vi "Measure.vi"(8 "error in (no error)":errorcluster, 11 "IV_meas in":refnum<class "IV_meas.lvclass">) -> (0 "error out":errorcluster, 1 "Current Value":dbl, 2 "Result":dbl, 3 "IV_meas out":refnum<class "IV_meas.lvclass">)   [LabVIEW 2018, in "IV_meas.lvclass"]
uses:
  IV_meas.lvclass
  Abstract/Measurement/Measurement2D/Measurement2D.lvclass
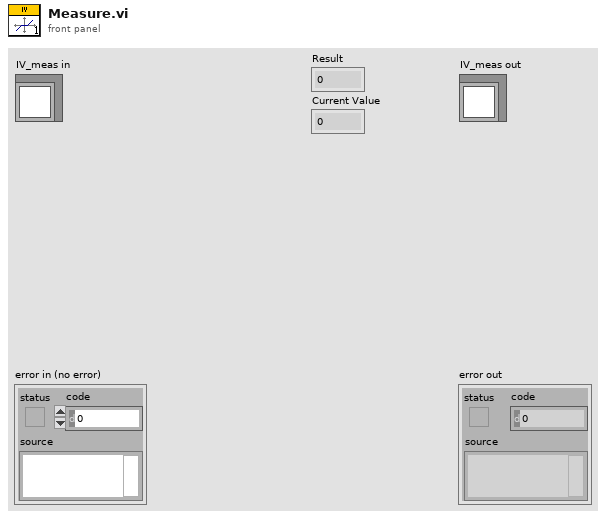
[diagram p1: front panel]
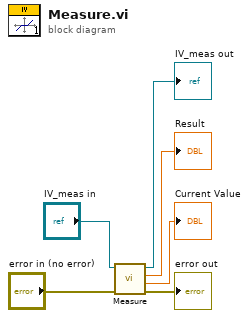
[diagram p0: block diagram]
diagram:
  n1 = call-parent "Measure.vi"("error in (no error)"="error in (no error)", "Measurement2D in"="IV_meas in") -> ("error out"=→"error out":errorcluster, "Current Value"=→"Current Value":dbl, "Result"=→"Result":dbl, "Measurement2D out"=→"IV_meas out":refnum<class "IV_meas.lvclass">)  [unwired: 6 in]
